vi "Get Log File Description.vi"(6 "timeout (ms)":i32=-1, 8 "error in (no error)":errorcluster, 11 "FlexLogger_gRPC in":refnum<class "FlexLogger_gRPC.lvclass">) -> (0 "error out":errorcluster, 2 "log_file_description":string, 3 "FlexLogger_gRPC out":refnum<class "FlexLogger_gRPC.lvclass">)   [LabVIEW 2020, in "FlexLogger_gRPC.lvlib" / "FlexLogger_gRPC.lvclass"]
doc: "Gets the data rate level of the subsystem that owns a channel."
uses:
  FlexLogger_gRPC.lvclass
  FlexLogger_client/RPC Messages/flexlogger_GetLogFileDescriptionRequest.ctl
  FlexLogger_client/RPC Messages/flexlogger_ElementIdentifier.ctl
  FlexLogger_gRPC.lvclass/FlexLogger_gRPC.ctl
  FlexLogger_client/FlexLogger_client.lvlib
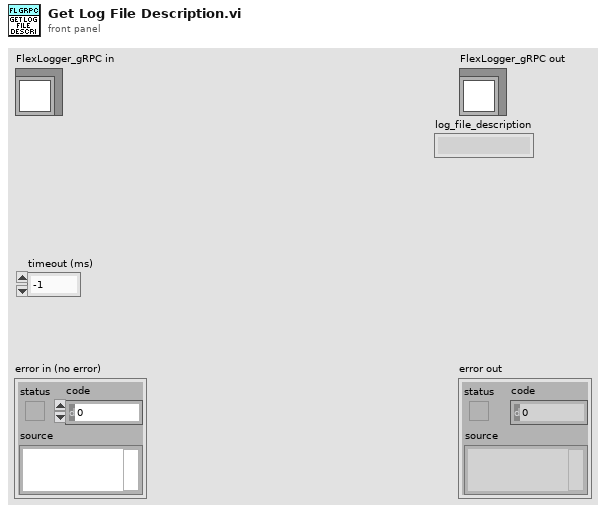
[diagram p1: front panel]
types:
  T1 = typedef "FlexLogger_client.lvlib/flexlogger_GetLogFileDescriptionRequest.ctl" = cluster{"document_identifier":T2}
  T2 = typedef "FlexLogger_client.lvlib/flexlogger_ElementIdentifier.ctl" = cluster{"project_id":string, "file_name":string, "element_id":string, "subpart_id":string}
  T3 = typedef "grpc-lvsupport-release.lvlib/grpcId.ctl" = u64
  T4 = typedef "FlexLogger_client.lvlib/flexlogger_GetLogFileDescriptionResponse.ctl" = cluster{"log_file_description":string}
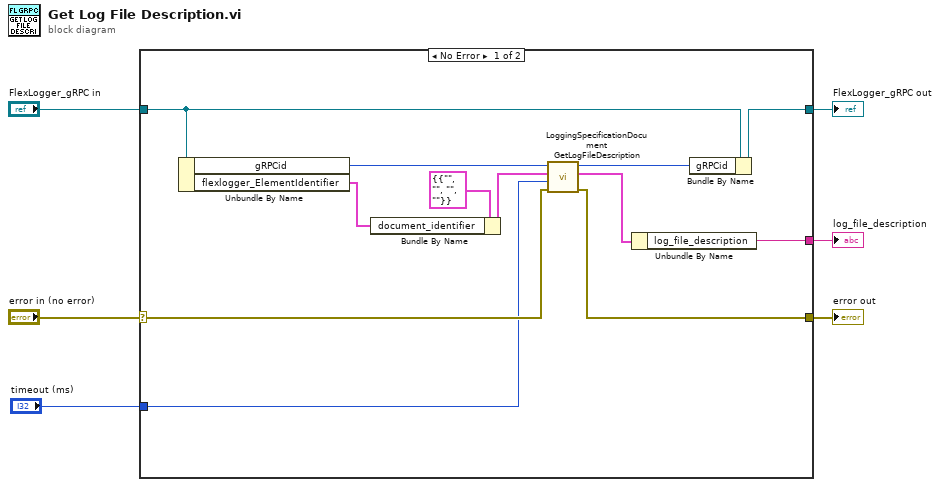
[diagram p0: block diagram]
diagram:
  n1 = case shown="No Error" "error in (no error)" {
    selector: "error in (no error)" -> [w14 w19]
    tunnel: "FlexLogger_gRPC in" -> [w18 w20]
    tunnel: [w17 w20] -> w6
    tunnel: [w13 w19] -> w4
    tunnel: "timeout (ms)" -> [w12 _]
    tunnel: [w7 _] -> w1
    frame No Error {
      n2 = Unbundle By Name(w18) -> ("gRPCid"=w16:T3, "flexlogger_ElementIdentifier"=w10:T2)
      n3 = Bundle By Name(cluster=T1 {"document_identifier"={"project_id"="", "file_name"="", "element_id"="", "subpart_id"=""}} ("Request Data"), "document_identifier"=w10) -> (w9:T1)
      n4 = call "LoggingSpecificationDocument GetLogFileDescription.vi"("error in"=w14, "timeout (ms)"=w12, "Request Data"=w9, "gRPC ID"=w16) -> ("error out"=w13:errorcluster, "Response Data"=w8:T4, "gRPC ID out"=w15:T3)  [unwired: 5 in]
      n5 = Unbundle By Name(w8) -> ("log_file_description"=w7:string)
      n6 = Bundle By Name(cluster=w18, "gRPCid"=w15) -> (w17:refnum<class "FlexLogger_gRPC.lvclass">)
    }
    frame Error {
    }
  }
  "error out" <- w4
  "FlexLogger_gRPC out" <- w6
  "log_file_description" <- w1
